vi "output_callback.vi"(4 "Output Event":refnum<user-event>, 5 "Event Data":cluster{"sender":refnum<k24>, "e":refnum<k24>}, 6 "Control Ref":refnum<k24>, 7 "Event Common Data":T1) -> ()   [LabVIEW 2013, in "dotnet_system_exec.lvclass"]
doc: "This vi is used to process the callback when data from a stream is available. Then sends that data out via a user event provided."
uses:
  dotnet_system_exec.lvclass
panel:
  out "String":string
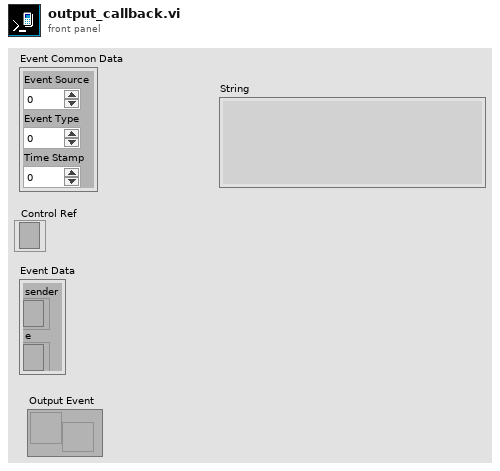
[diagram p1: front panel]
types:
  T1 = cluster{"Event Source":i32, "Event Type":u32, "Time Stamp":u32}
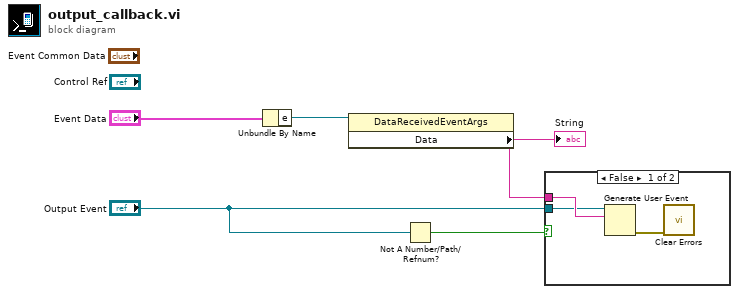
[diagram p0: block diagram]
diagram:
  n1 = Unbundle By Name("Event Data") -> ("e"=w5:refnum<k24>)
  n2 = property class="DataReceivedEventArgs"(reference=w5) -> ("Data"=w3:string)  [unwired: 1 in, 2 out]
  "String" <- w3
  n3 = Not A Number/Path/Refnum?(number/path/refnum="Output Event") -> (NaN/Path/Refnum?=w1:bool)
  n4 = case shown="False" w1 {
    tunnel: w3 -> [w8 _]
    tunnel: "Output Event" -> [w7 _]
    frame False {
      n5 = Generate User Event(user event=w7, event data cluster=w8) -> (error out=w6:errorcluster)  [unwired: 2 in, 1 out]
      n6 = call <vilib>:"Clear Errors.vi"("error in (no error)"=w6) -> ()  [unwired: 5 in, 2 out]
    }
    frame True {
    }
  }
